vi "Log AO.vi"(8 "error in (no error)":errorcluster, 11 "Instrument.Lockin in":refnum<class "Instrument.Lockin.lvclass">) -> (0 "error out":errorcluster, 3 "Instrument.Lockin out":refnum<class "Instrument.Lockin.lvclass">)   [LabVIEW 2019, in "Instrument.Lockin.lvlib" / "Instrument.Lockin.lvclass"]
uses:
  Instrument.Lockin.lvclass
  C:/Program Files/National Instruments/LabVIEW 2019/user.lib/LevyLab/Instrument Framework/Instrument/Instrument.lvclass
  Instrument.Lockin.lvclass/Instrument.Lockin.ctl
  <userlib>/LevyLab/Instrument Framework/Instrument/Instrument.lvclass
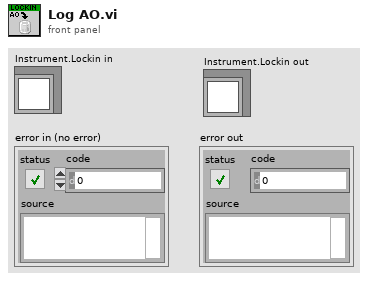
[diagram p1: front panel]
types:
  T1 = typedef "Instrument.Lockin.lvlib/Instrument.Lockin.lvclass/Lockin.LogSweepAOAI--Cluster.ctl" = cluster{"ChassisSerialNumber":u32, "Channel":i32, "Data":dbl, "Sweeping?":bool}
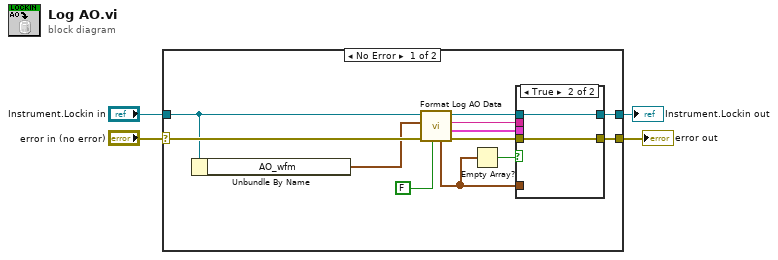
[diagram p0: block diagram]
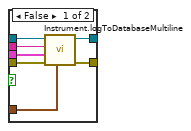
[diagram p2: hidden frame]
diagram:
  n1 = case shown="No Error" "error in (no error)" {
    selector: "error in (no error)" -> [w15 w27]
    tunnel: "Instrument.Lockin in" -> [w14 w26]
    tunnel: [w16 w27] -> w3
    tunnel: [w13 w26] -> w1
    frame No Error {
      n2 = Unbundle By Name(w14) -> ("AO_wfm"=w12:waveform(dbl)[])
      n3 = call "Format Log AO Data.vi"("Sweeping?"=FALSE, "error in (no error)"=w15, "waveform"=w12, "Instrument.Lockin in"=w14) -> ("error out"=w7:errorcluster, "Log Data"=w9:T1[], "Log Paths"=w10:string, "Instrument.Lockin out"=w11:refnum<class "Instrument.Lockin.lvclass">, "Times"=w5:timestamp[])  [unwired: 3 in]
      n4 = Empty Array?(array=w5) -> (empty?=w6:bool)
      n5 = case shown="True" w6 {
        tunnel: [w23 w25] -> w16
        tunnel: [w22 w24] -> w13
        tunnel: w11 -> [w21 w24]
        tunnel: w10 -> [w20 _]
        tunnel: w9 -> [w19 _]
        tunnel: w5 -> [w18 _]
        tunnel: w7 -> [w17 w25]
        frame False {
          n6 = call <userlib>:"Instrument.logToDatabaseMultiline.vi"("timestamps"=w18, "error in (no error)"=w17, "Data"=w19, "Paths"=w20, "Instrument"=w21) -> ("error out"=w23:errorcluster, "Instrument out"=w22:refnum<class "Instrument.Lockin.lvclass">)  [unwired: 5 in]
        }
        frame True {
        }
      }
    }
    frame Error {
    }
  }
  "error out" <- w3
  "Instrument.Lockin out" <- w1
